vi "stream_dataC25_CodEscape.vi"(6 "Offsets":dbl[](array[numeric]), 7 "Gains":dbl[](array[numeric]), 8 "error out 2":errorcluster, 11 "VISA resource name out 2":refnum<visa-resource-name>) -> (0 "VISA resource name out":refnum<visa-resource-name>, 1 "DATA":dbl, 2 "P-Channel":i32, 3 "N-channel":i32, 4 "NumChannel":i32, 5 "NumBytes":i32, 9 "Gain":i32, 10 "error out":errorcluster)   [LabVIEW 2011]
panel:
  out "(hi.lo)":i16
  out "Data 2":i32
  out "Data 1":i32
  out "NumCommand":i32
  out "CRC":i16
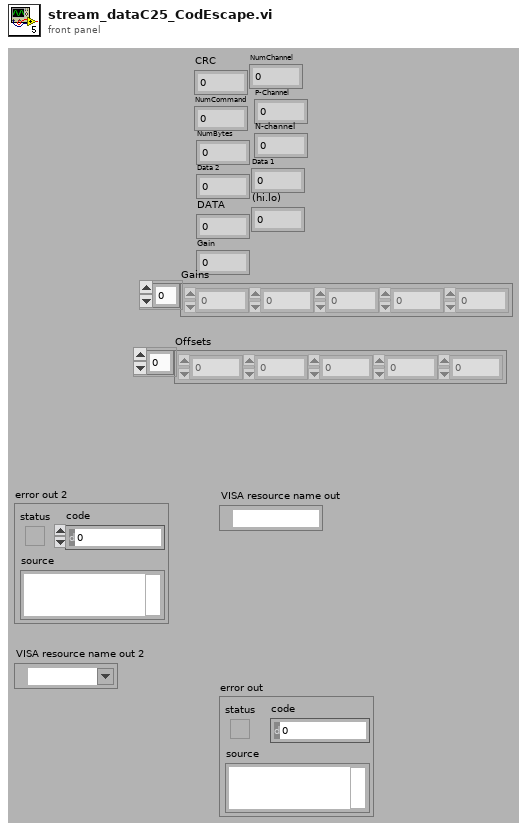
[diagram p1: front panel]
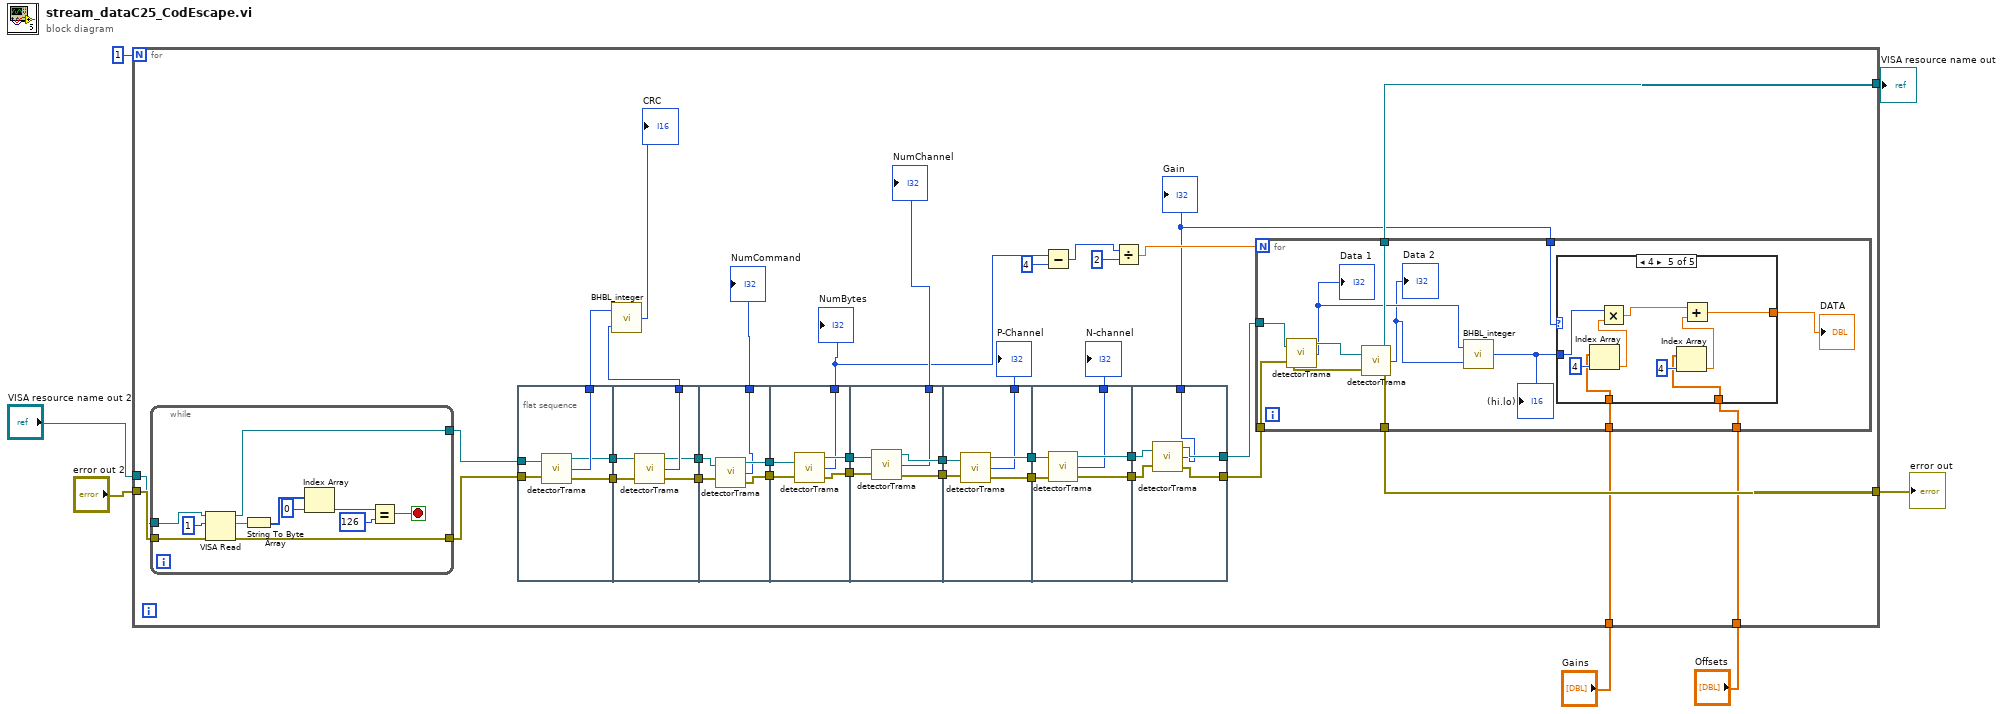
[diagram p0: block diagram]
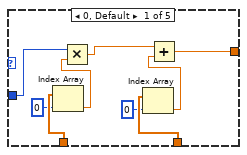
[diagram p2: hidden frame]
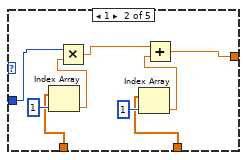
[diagram p3: hidden frame]
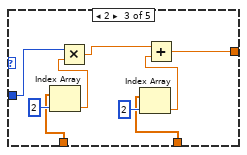
[diagram p4: hidden frame]
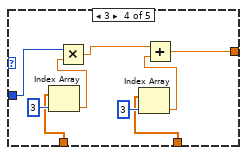
[diagram p5: hidden frame]
diagram:
  n1 = for {
    N: 1 -> [_]
    tunnel: "error out 2" -> [w44]
    tunnel: "VISA resource name out 2" -> [w43]
    tunnel: [w20] -> w5
    tunnel: [w19] -> w4
    tunnel: "Gains" -> [w9]
    tunnel: "Offsets" -> [w8]
    n2 = while {
      tunnel: w43 -> [w146]
      tunnel: w44 -> [w147]
      tunnel: [w144] -> w42
      tunnel: [w143] -> w41
      stop <- w148 stop-if-true
      n3 = VISA Read(VISA resource name=w146, byte count=u32 1, error in (no error)=w147) -> (VISA resource name out=w144:refnum<visa-resource-name>, read buffer=w153:string, error out=w143:errorcluster)  [unwired: 1 out]
      n4 = String To Byte Array(string=w153) -> (unsigned byte array=w152:u8[])
      n5 = Index Array(array=w152, index=0) -> (element=w150:u8)
      n6 = Equal?(x=w150, y=u8 126) -> (x = y?=w148:bool)
    }
    n7 = flat-sequence {
      tunnel: w42 -> [w107]
      tunnel: w41 -> [w106]
      tunnel: [w105] -> w28
      tunnel: [w104] -> w40
      tunnel: [w103] -> w39
      tunnel: w40 -> [w112]
      tunnel: w39 -> [w111]
      tunnel: [w110] -> w27
      tunnel: [w109] -> w38
      tunnel: [w108] -> w37
      tunnel: w38 -> [w117]
      tunnel: w37 -> [w116]
      tunnel: [w115] -> w36
      tunnel: [w114] -> w35
      tunnel: [w113] -> w25
      tunnel: w36 -> [w122]
      tunnel: w35 -> [w121]
      tunnel: [w120] -> w34
      tunnel: [w119] -> w33
      tunnel: [w118] -> w18
      tunnel: w34 -> [w127]
      tunnel: w33 -> [w126]
      tunnel: [w125] -> w32
      tunnel: [w124] -> w31
      tunnel: [w123] -> w24
      tunnel: w32 -> [w132]
      tunnel: w31 -> [w131]
      tunnel: [w130] -> w30
      tunnel: [w129] -> w29
      tunnel: [w128] -> w23
      tunnel: w30 -> [w137]
      tunnel: w29 -> [w136]
      tunnel: [w133] -> w22
      tunnel: [w135] -> w16
      tunnel: [w134] -> w15
      tunnel: [w139] -> w21
      tunnel: [w140] -> w14
      tunnel: w16 -> [w142]
      tunnel: w15 -> [w141]
      tunnel: [w138] -> w10
      frame #0 {
        n8 = call "detectorTrama.vi"("VISA resource name"=w107, "error in (no error)"=w106) -> ("VISA resource name 2"=w104:refnum<visa-resource-name>, "Numeric"=w105:i32, "error in (no error) 2"=w103:errorcluster)
      }
      frame #1 {
        n9 = call "detectorTrama.vi"("VISA resource name"=w112, "error in (no error)"=w111) -> ("VISA resource name 2"=w109:refnum<visa-resource-name>, "Numeric"=w110:i32, "error in (no error) 2"=w108:errorcluster)
      }
      frame #2 {
        n10 = call "detectorTrama.vi"("VISA resource name"=w117, "error in (no error)"=w116) -> ("VISA resource name 2"=w115:refnum<visa-resource-name>, "Numeric"=w113:i32, "error in (no error) 2"=w114:errorcluster)
      }
      frame #3 {
        n11 = call "detectorTrama.vi"("VISA resource name"=w122, "error in (no error)"=w121) -> ("VISA resource name 2"=w120:refnum<visa-resource-name>, "Numeric"=w118:i32, "error in (no error) 2"=w119:errorcluster)
      }
      frame #4 {
        n12 = call "detectorTrama.vi"("VISA resource name"=w127, "error in (no error)"=w126) -> ("VISA resource name 2"=w125:refnum<visa-resource-name>, "Numeric"=w123:i32, "error in (no error) 2"=w124:errorcluster)
      }
      frame #5 {
        n13 = call "detectorTrama.vi"("VISA resource name"=w132, "error in (no error)"=w131) -> ("VISA resource name 2"=w130:refnum<visa-resource-name>, "Numeric"=w128:i32, "error in (no error) 2"=w129:errorcluster)
      }
      frame #6 {
        n14 = call "detectorTrama.vi"("VISA resource name"=w137, "error in (no error)"=w136) -> ("VISA resource name 2"=w135:refnum<visa-resource-name>, "Numeric"=w133:i32, "error in (no error) 2"=w134:errorcluster)
      }
      frame #7 {
        n15 = call "detectorTrama.vi"("VISA resource name"=w142, "error in (no error)"=w141) -> ("VISA resource name 2"=w140:refnum<visa-resource-name>, "Numeric"=w138:i32, "error in (no error) 2"=w139:errorcluster)
      }
    }
    n16 = call "BHBL_integer.vi"("lo(x)"=w27, "hi(x)"=w28) -> ("(hi.lo)"=→"CRC":i16)
    n17 = Subtract(x=w18, y=4) -> (x-y=w13:i32)
    n18 = Divide(x=w13, y=2) -> (x/y=w12:dbl)
    n19 = for {
      N: w12 -> [_]
      tunnel: w14 -> [w57]
      tunnel: w21 -> [w56]
      tunnel: [w53] -> w20
      tunnel: [w52] -> w19
      tunnel: w10 -> [w48]
      tunnel: w9 -> [w47]
      tunnel: w8 -> [w46]
      n20 = call "detectorTrama.vi"("VISA resource name"=w57, "error in (no error)"=w56) -> ("VISA resource name 2"=w55:refnum<visa-resource-name>, "Numeric"=w51:i32, "error in (no error) 2"=w54:errorcluster)
      "Data 1" <- w51
      n21 = call "detectorTrama.vi"("VISA resource name"=w55, "error in (no error)"=w54) -> ("VISA resource name 2"=w53:refnum<visa-resource-name>, "Numeric"=w50:i32, "error in (no error) 2"=w52:errorcluster)
      "Data 2" <- w50
      n22 = call "BHBL_integer.vi"("lo(x)"=w50, "hi(x)"=w51) -> ("(hi.lo)"=w49:i16)
      "(hi.lo)" <- w49
      n23 = case shown="4" w48 {
        tunnel: w49 -> [w62 w69 w76 w85 w94]
        tunnel: w47 -> [w66 w68 w77 w86 w95]
        tunnel: w46 -> [w64 w67 w78 w87 w96]
        tunnel: [w58 w70 w79 w88 w97] -> w45
        frame 0, Default {
          n24 = Index Array(array=w66, index=0) -> (element=w61:dbl)
          n25 = Multiply(x=w62, y=w61) -> (x*y=w60:dbl)
          n26 = Index Array(array=w64, index=0) -> (element=w59:dbl)
          n27 = Add(x=w60, y=w59) -> (x+y=w58:dbl)
        }
        frame 1 {
          n28 = Index Array(array=w68, index=1) -> (element=w73:dbl)
          n29 = Multiply(x=w69, y=w73) -> (x*y=w72:dbl)
          n30 = Index Array(array=w67, index=1) -> (element=w71:dbl)
          n31 = Add(x=w72, y=w71) -> (x+y=w70:dbl)
        }
        frame 2 {
          n32 = Index Array(array=w77, index=2) -> (element=w82:dbl)
          n33 = Multiply(x=w76, y=w82) -> (x*y=w81:dbl)
          n34 = Index Array(array=w78, index=2) -> (element=w80:dbl)
          n35 = Add(x=w81, y=w80) -> (x+y=w79:dbl)
        }
        frame 3 {
          n36 = Index Array(array=w86, index=3) -> (element=w91:dbl)
          n37 = Multiply(x=w85, y=w91) -> (x*y=w90:dbl)
          n38 = Index Array(array=w87, index=3) -> (element=w89:dbl)
          n39 = Add(x=w90, y=w89) -> (x+y=w88:dbl)
        }
        frame 4 {
          n40 = Index Array(array=w95, index=4) -> (element=w100:dbl)
          n41 = Multiply(x=w94, y=w100) -> (x*y=w99:dbl)
          n42 = Index Array(array=w96, index=4) -> (element=w98:dbl)
          n43 = Add(x=w99, y=w98) -> (x+y=w97:dbl)
        }
      }
      "DATA" <- w45
    }
    "NumCommand" <- w25
    "NumBytes" <- w18
    "NumChannel" <- w24
    "P-Channel" <- w23
    "N-channel" <- w22
    "Gain" <- w10
  }
  "VISA resource name out" <- w5
  "error out" <- w4
